vi "ArduinoSerialTest3.vi"() -> ()   [LabVIEW 2013]
uses:
  <vilib>/Instr/_visa.llb/VISA Configure Serial Port (Instr).vi
panel:
  out "Serial Response":string
  in  "Invert Direction":bool
  in  "Motor Name":dbl
  in  "Resolution":T1(radio)
  in  "-90":bool
  in  "-270":bool
  in  "-180":bool
  in  "-360":bool
  in  "+360":bool
  out "Auto":dbl
  in  "+180":bool
  in  "+270":bool
  in  "+90":bool
  in  "Manual":dbl
  in  "stop":bool
  in  "Go":bool
  in  "VISA resource name":refnum<visa-resource-name>="COM8"
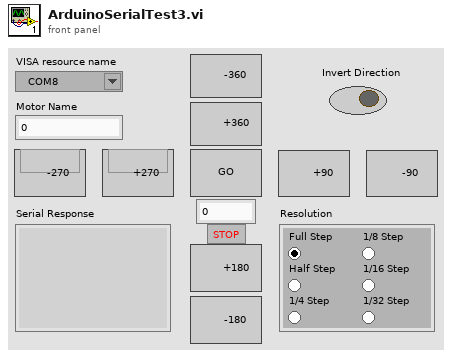
[diagram p1: front panel]
types:
  T1 = enum32{"Full Step", "Half Step", "1/4 Step", "1/8 Step", "1/16 Step", "1/32 Step"}
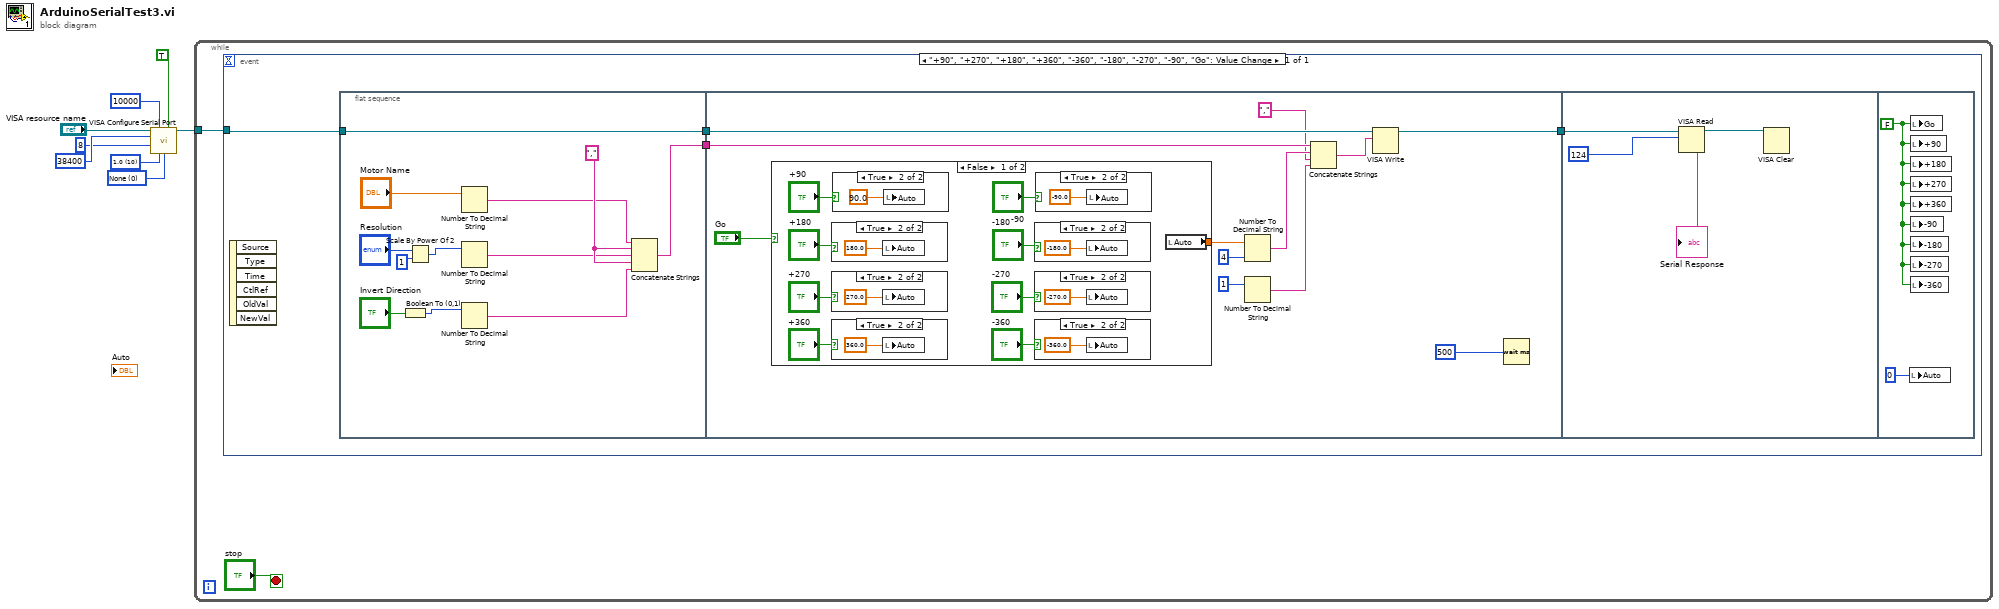
[diagram p0: block diagram]
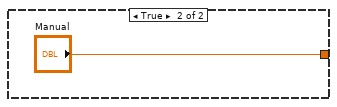
[diagram p10: hidden frame]
diagram:
  w3 = u16 0 items=["None", "XON/XOFF", "RTS/CTS", "XON/XOFF & RTS/CTS", "DTR/DSR", "XON/XOFF & DTR/DSR"] ("flow control (0:none)")
  w4 = u16 10 items=["1.0"=10, "1.5"=15, "2.0"=20] ("stop bits (10: 1 bit)")
  n1 = call-poly "VISA Configure Serial Port"("VISA resource name"="VISA resource name", "timeout (10sec)"=u32 10000, "Enable Termination\nChar (T)"=TRUE ("Enable Termination\nChar (T)"), "baud rate (9600)"=u32 38400, "data bits (8)"=u16 8, "stop bits (10: 1 bit)"=w4, "flow control (0:none)"=w3) -> ("VISA resource name out"=w8:refnum<visa-resource-name>)  [unwired: 7 in, 1 out]
  n2 = while {
    tunnel: w8 -> [w10]
    stop <- "stop" stop-if-true
    n3 = event shown="[0] \"+90\", \"+270\", \"+180\", \"+360\", \"-360\", \"-180\", \"-270\", \"-90\", \"Go\": Value Change" {
      selector: _ -> [_]
      dyn-events: _ -> [_]
      timeout: _ -> [_]
      tunnel: w10 -> [w14]
      event "+90", "+270", "+180", "+360", "-360", "-180", "-270", "-90", "Go": Value Change {
        n4 = event-data() -> ()  [unwired: 1 in, 6 out]
        n5 = flat-sequence {
          tunnel: w14 -> [w26]
          tunnel: [w26] -> w13
          tunnel: [w15] -> w12
          tunnel: w13 -> [w31]
          tunnel: w12 -> [w32]
          tunnel: [w30] -> w11
          tunnel: w11 -> [w60]
          frame #0 {
            w19 = ","
            n6 = Boolean To (0,1)(Boolean="Invert Direction") -> (0, 1=w21:i16)
            n7 = Scale By Power Of 2(n="Resolution", x=1) -> (x*2^n=w20:i32)
            n8 = Number To Decimal String(number="Motor Name") -> (decimal integer string=w18:string)  [unwired: 1 in]
            n9 = Number To Decimal String(number=w20) -> (decimal integer string=w17:string)  [unwired: 1 in]
            n10 = Number To Decimal String(number=w21) -> (decimal integer string=w16:string)  [unwired: 1 in]
            n11 = Concatenate Strings(w18, w19, w17, w19, w16) -> (w15:string)
          }
          frame #1 {
            n12 = case shown="False" "Go" {
              tunnel: [w44 "Manual"] -> w33
              frame False {
                n13 = case shown="True" "+180" {
                  frame False {
                  }
                  frame True {
                    n14 = local write "Auto"(180.0 ("Numeric")) -> ()
                  }
                }
                n15 = case shown="True" "+270" {
                  frame False {
                  }
                  frame True {
                    n16 = local write "Auto"(270.0 ("Numeric")) -> ()
                  }
                }
                n17 = case shown="True" "+360" {
                  frame False {
                  }
                  frame True {
                    n18 = local write "Auto"(360.0 ("Numeric")) -> ()
                  }
                }
                n19 = case shown="True" "+90" {
                  frame False {
                  }
                  frame True {
                    n20 = local write "Auto"(90.0 ("Numeric")) -> ()
                  }
                }
                n21 = case shown="True" "-180" {
                  frame False {
                  }
                  frame True {
                    n22 = local write "Auto"(-180.0 ("Numeric")) -> ()
                  }
                }
                n23 = case shown="True" "-270" {
                  frame False {
                  }
                  frame True {
                    n24 = local write "Auto"(-270.0 ("Numeric")) -> ()
                  }
                }
                n25 = case shown="True" "-360" {
                  frame False {
                  }
                  frame True {
                    n26 = local write "Auto"(-360.0 ("Numeric")) -> ()
                  }
                }
                n27 = case shown="True" "-90" {
                  frame False {
                  }
                  frame True {
                    n28 = local write "Auto"(-90.0 ("Numeric")) -> ()
                  }
                }
                n29 = local read "Auto"() -> (w44:dbl)
              }
              frame True {
              }
            }
            n30 = Number To Decimal String(number=w33, width (-)=4) -> (decimal integer string=w36:string)
            n31 = Number To Decimal String(number=1) -> (decimal integer string=w28:string)  [unwired: 1 in]
            n32 = Concatenate Strings(w32, w36, ",", w28) -> (w37:string)
            n33 = VISA Write(VISA resource name=w31, write buffer=w37) -> (VISA resource name out=w30:refnum<visa-resource-name>)  [unwired: 1 in, 2 out]
            n34 = Wait (ms)(milliseconds to wait=u32 500) -> ()  [unwired: 1 out]
          }
          frame #2 {
            n35 = VISA Read(VISA resource name=w60, byte count=u32 124) -> (VISA resource name out=w57:refnum<visa-resource-name>, read buffer=→"Serial Response":string)  [unwired: 1 in, 2 out]
            n36 = VISA Clear(VISA resource name=w57) -> ()  [unwired: 1 in, 2 out]
          }
          frame #3 {
            w61 = FALSE
            n37 = local write "Auto"(0) -> ()
            n38 = local write "Go"(w61) -> ()
            n39 = local write "+90"(w61) -> ()
            n40 = local write "+180"(w61) -> ()
            n41 = local write "+270"(w61) -> ()
            n42 = local write "+360"(w61) -> ()
            n43 = local write "-90"(w61) -> ()
            n44 = local write "-180"(w61) -> ()
            n45 = local write "-270"(w61) -> ()
            n46 = local write "-360"(w61) -> ()
          }
        }
      }
    }
  }
